vi "octave_close.vi"(7 "timeout [ms]":i32, 8 "error in":errorcluster, 10 "try kill if error":bool=TRUE, 11 "instance handle in":u32[](array[numeric])) -> (0 "error out":errorcluster, 1 "failed":bool, 2 "exit code":i32, 3 "instance handle out":u32[](array[numeric]))   [LabVIEW 2011]
doc: "Tries to terminate GNU Octave process instance. First it sends 'exit' command and waits if Octave responds. If this fails and used has allowed hard process kill (TerminateProcess() WinAPI) it tries to kill it. Both tries have timeouts. If zero timeout is set it waits for ever so it can hangup! \nIf Octave is successfully terminated process instance handle memory is freed so no other VI can access closed process/pipes handles.\nIf no process instance handle is connected, last one from global variable is used or new instance handle is stored to it."
uses:
  octave_var.vi
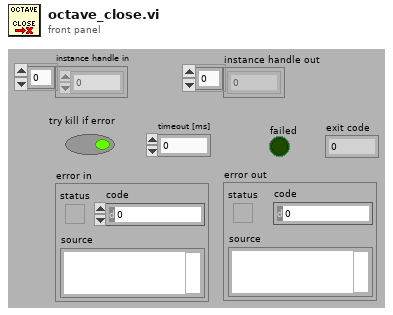
[diagram p1: front panel]
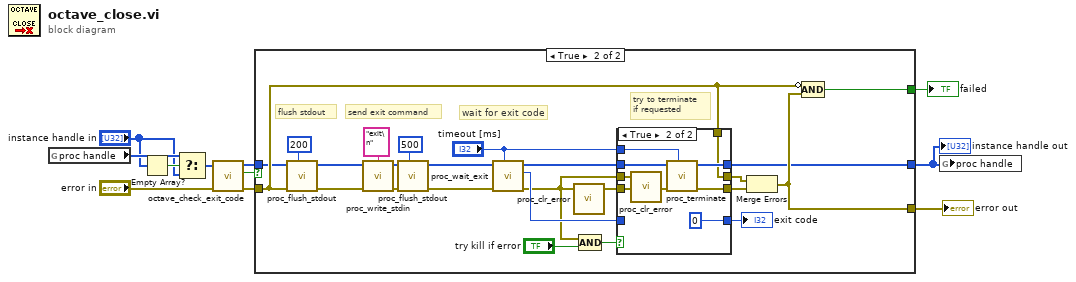
[diagram p0: block diagram]
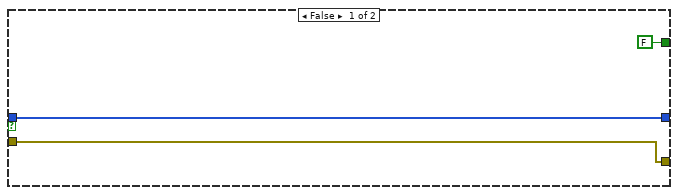
[diagram p2: hidden frame]
diagram:
  n1 = global read "octave_var.vi" "proc handle"() -> (w11:u32[])
  n2 = Empty Array?(array="instance handle in") -> (empty?=w10:bool)
  n3 = Select(t=w11, s=w10, f="instance handle in") -> (s? t:f=w5:u32[])
  n4 = call "octave_check_exit_code.vi"("error in"="error in", "instance handle in"=w5) -> ("error out"=w6:errorcluster, "running"=w3:bool, "instance handle out"=w4:u32[])  [unwired: 5 in, 2 out]
  n5 = case shown="True" w3 {
    tunnel: [w14 w16] -> w8
    tunnel: w6 -> [w13 w19]
    tunnel: w4 -> [w14 w18]
    tunnel: [w13 w17] -> w2
    tunnel: [FALSE w15] -> w1
    frame False {
    }
    frame True {
      # "flush stdout"
      # "try to terminate\nif requested"
      # "wait for exit code"
      # "send exit command"
      n6 = call "proc_flush_stdout.vi"("interval [ms]"=200, "error in"=w19, "process instance handle in"=w18) -> ("error out"=w27:errorcluster, "process instance handle out"=w26:u32[])  [unwired: 6 in, 1 out]
      n7 = call "proc_write_stdin.vi"("error in"=w27, "write buffer"="exit\n", "process instance handle in"=w26) -> ("error out"=w23:errorcluster, "process instance handle out"=w20:u32[])  [unwired: 6 in, 1 out]
      n8 = call "proc_flush_stdout.vi"("interval [ms]"=500, "error in"=w23, "process instance handle in"=w20) -> ("error out"=w22:errorcluster, "process instance handle out"=w21:u32[])  [unwired: 6 in, 1 out]
      n9 = call "proc_wait_exit.vi"("timeout [ms]"="timeout [ms]", "error in"=w22, "process instance handle in"=w21) -> ("error out"=w30:errorcluster, "exit code"=w32:i32, "process instance handle out"=w35:u32[])  [unwired: 6 in]
      n10 = call "proc_clr_error.vi"("error in (no error)"=w30) -> ("error out"=w38:errorcluster)  [unwired: 4 in]
      n11 = Compound Arithmetic op=AND(w30, "try kill if error") -> (w36:bool)
      n12 = case shown="True" w36 {
        tunnel: [w42 w47] -> w34
        tunnel: w38 -> [w42 w50]
        tunnel: [w41 w49] -> w16
        tunnel: w35 -> [w41 w48]
        tunnel: w32 -> [w40 _]
        tunnel: [w40 0 ("exit code")] -> w33
        tunnel: w30 -> [w39 w44]
        tunnel: [w39 w45] -> w31
        tunnel: w19 -> [_ w45]
        tunnel: "timeout [ms]" -> [_ w43]
        frame False {
        }
        frame True {
          n13 = call "proc_clr_error.vi"("error in (no error)"=w44) -> ()  [unwired: 4 in, 1 out]
          n14 = call "proc_terminate.vi"("timeout [ms]"=w43, "error in"=w50, "process instance handle in"=w48) -> ("error out"=w47:errorcluster, "process instance handle out"=w49:u32[])  [unwired: 7 in]
        }
      }
      "exit code" <- w33
      n15 = Merge Errors(w31, w34) -> (w17:errorcluster)
      n16 = Compound Arithmetic op=AND(invert w19, w17) -> (w15:bool)
    }
  }
  "instance handle out" <- w8
  "error out" <- w2
  "failed" <- w1
  n17 = global write "octave_var.vi" "proc handle"(w8) -> ()
